vi "SERIAL_AHRSPosGlobal.vi"(10 "Set":bool=TRUE, 11 "AHRSPos Data":T1) -> (3 "AHRSPos Data":T1)   [LabVIEW 2014, in "navX-MXP IMU.lvlib"]
uses:
  navX-MXP IMU.lvlib
  TypeDefs/navX AHRSPos Data.ctl
  COMMON/TypeDefs/Data TypeDefs/navX Quaternion Data.ctl
  COMMON/TypeDefs/Data TypeDefs/navX Vector Data.ctl
  <vilib>/Rock Robotics/SystemInterfaces/Utilities/FPGA_UtilitiesRead LocalTime.vi
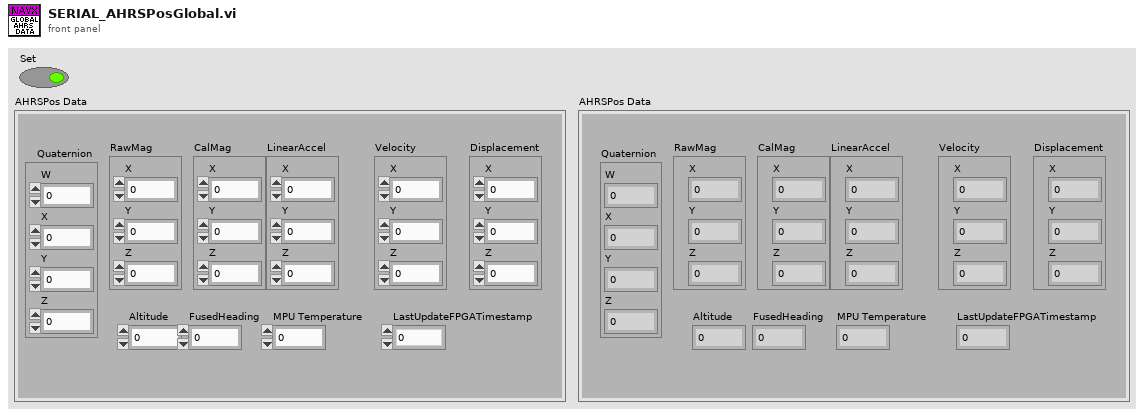
[diagram p1: front panel]
types:
  T1 = typedef "navX-MXP IMU.lvlib/navX AHRSPos Data.ctl" = cluster{"Quaternion":T2, "RawMag":T3, "CalMag":T3, "LinearAccel":T3, "Displacement":T3, "Velocity":T3, "Altitude":dbl, "FusedHeading":dbl, "MPU Temperature":dbl, "LastUpdateFPGATimestamp":dbl}
  T2 = typedef "navX-MXP IMU.lvlib/navX Quaternion Data.ctl" = cluster{"W":dbl, "X":dbl, "Y":dbl, "Z":dbl}
  T3 = typedef "navX-MXP IMU.lvlib/navX Vector Data.ctl" = cluster{"X":dbl, "Y":dbl, "Z":dbl}
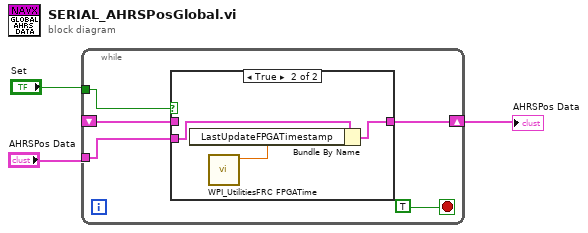
[diagram p0: block diagram]
diagram:
  n1 = while {
    shift-right: [w5] -> w1
    shift-left: _ -> [w4]
    tunnel: "AHRSPos Data" -> [w6]
    tunnel: "Set" -> [w7]
    stop <- TRUE stop-if-true
    n2 = case shown="True" w7 {
      tunnel: w6 -> [_ w12]
      tunnel: [w9 w10] -> w5
      tunnel: w4 -> [w9 _]
      frame False {
      }
      frame True {
        n3 = call <vilib>:"WPI_UtilitiesFRC FPGATime.vi"() -> ("FPGA Time"=w11:dbl)  [unwired: 10 in, 1 out]
        n4 = Bundle By Name(cluster=w12, "LastUpdateFPGATimestamp"=w11) -> (w10:T1)
      }
    }
  }
  "AHRSPos Data" <- w1
